vi "Create File Paths.vi"(8 "error in (no error)":errorcluster) -> (0 "error out":errorcluster)   [LabVIEW 2012]
doc: "Initializes file paths for the system:\nIni path - Path to ini file that contains system settings\nPattern filepath - path to the matlab generated pattern files\nArena Config Filepath - path to the arena configuration files that designate the panel to bus matching"
uses:
  HHMI - Filepaths global.vi
  Common/File IO/FileIO lib.lvlib
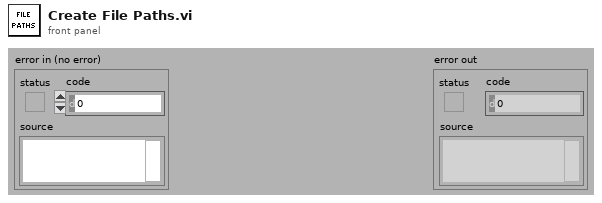
[diagram p1: front panel]
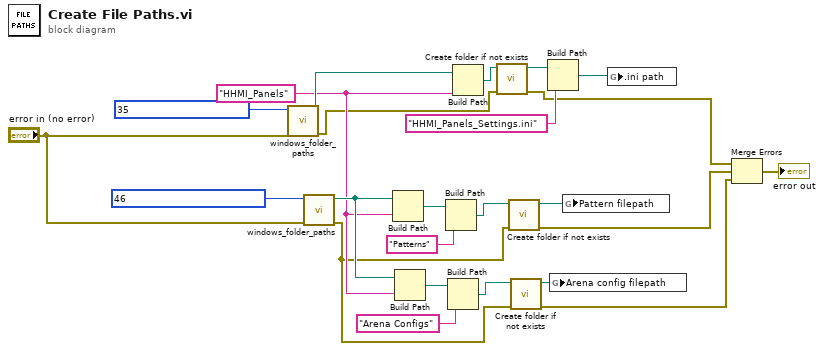
[diagram p0: block diagram]
diagram:
  w7 = "HHMI_Panels" ("name or relative path")
  n1 = call "windows_folder_paths.vi"("error in (no error)"="error in (no error)", "Folder Role"=35) -> ("error out"=w6:errorcluster, "System Folder Path"=w23:path)  [unwired: 8 out]
  n2 = call "windows_folder_paths.vi"("error in (no error)"="error in (no error)", "Folder Role"=46) -> ("error out"=w5:errorcluster, "System Folder Path"=w8:path)  [unwired: 8 out]
  n3 = Build Path(base path=w8, name or relative path=w7) -> (appended path=w17:path)
  n4 = Build Path(base path=w8, name or relative path=w7) -> (appended path=w9:path)
  n5 = Build Path(base path=w17, name or relative path="Patterns") -> (appended path=w15:path)
  n6 = Build Path(base path=w9, name or relative path="Arena Configs") -> (appended path=w11:path)
  n7 = Build Path(base path=w23, name or relative path=w7) -> (appended path=w21:path)
  n8 = call "Create folder if not exists.vi"("error in"=w6, "Path in"=w21) -> ("error out"=w4:errorcluster, "Path In"=w20:path)  [unwired: 7 in, 1 out]
  n9 = call "Create folder if not exists.vi"("error in"=w5, "Path in"=w15) -> ("error out"=w3:errorcluster, "Path In"=w14:path)  [unwired: 7 in, 1 out]
  n10 = call "Create folder if not exists.vi"("error in"=w5, "Path in"=w11) -> ("error out"=w2:errorcluster, "Path In"=w12:path)  [unwired: 7 in, 1 out]
  n11 = Build Path(base path=w20, name or relative path="HHMI_Panels_Settings.ini") -> (appended path=w18:path)
  n12 = global write "HHMI - Filepaths global.vi" "Arena config filepath"(w12) -> ()
  n13 = global write "HHMI - Filepaths global.vi" "Pattern filepath"(w14) -> ()
  n14 = global write "HHMI - Filepaths global.vi" ".ini path"(w18) -> ()
  n15 = Merge Errors(w4, w3, w2) -> (→"error out":errorcluster)
